vi "Config.vi"(8 "error in (no error)":errorcluster, 10 "Setting":variant, 11 "NI-Sync in":refnum<class "NI-Sync.lvclass">) -> (0 "error out":errorcluster, 3 "NI-Sync out":refnum<class "NI-Sync.lvclass">)   [LabVIEW 2025, in "Synchronization.lvlib" / "NI-Sync.lvclass"]
uses:
  NI-Sync.lvclass
  C:/Users/Public/Documents/Sandia National Labs/TSS Plugin/CEF.lvlibp/Node/CEF_Node.lvclass
  C:/Working copy/tss/Plugin/Engines/Synchronization/Synchronization Instrument/Synchronization Instrument.lvclass
  Synchronization configuration/Synchronization configuration.lvclass
  Synchronization configuration/Synchronization configuration.lvclass/Synchronization configuration.ctl
  NI-Sync.lvclass/NI-Sync.ctl
  Synchronization Channel/Synchronization Channel.lvclass
  Synchronization Channel configuration/Synchronization Channel configuration.lvclass
  C:/Users/Public/Documents/Sandia National Labs/TSS Plugin/Abstract Engine.lvlibp/Plugin/Abstract/Channel configuration/Channel configuration.lvclass
  Synchronization Channel configuration/Synchronization Channel configuration.lvclass/Synchronization Channel configuration.ctl
  Synchronization Channel configuration/Read Sync Channel Setting.vi
  Synchronization configuration/Read Sync Instrument Setting.vi
  Users/Public/Documents/Sandia National Labs/TSS Plugin/CEF.lvlibp/Node/ReadChildren.vi
  Users/Public/Documents/Sandia National Labs/TSS Plugin/Abstract Engine.lvlibp/Plugin/Abstract/Channel configuration/Read Channel Setting.vi
  Users/Public/Documents/Sandia National Labs/TSS Plugin/CEF.lvlibp/Node/CEF_Node.lvclass
  Users/Public/Documents/Sandia National Labs/TSS Plugin/CEF.lvlibp/serializable configuration/CEF_serializable configuration.lvclass
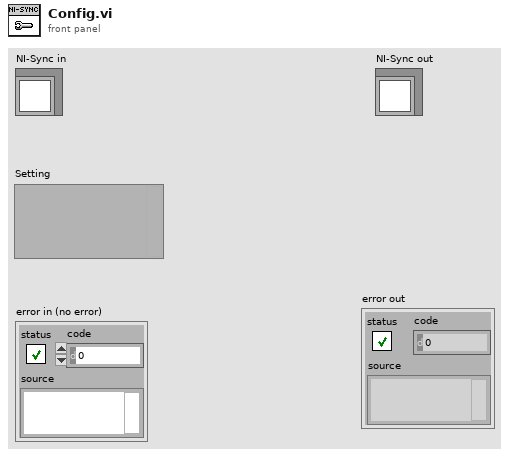
[diagram p1: front panel]
types:
  T1 = typedef "Synchronization.lvlib/Synchronization configuration.lvclass/Sync Instrument Setting.ctl" = cluster{"Synchronization Clock":string, "DDS Clock":dbl, "SyncDivide1":string, "SyncDivide2":string}
  T2 = typedef "Synchronization.lvlib/Synchronization Channel configuration.lvclass/Sync Channel Setting.ctl" = cluster{"Inverter":bool, "Update Edge":string, "Source":string, "Type":string, "Synchronization Clock":string, "Destination":string}
  T3 = typedef "Abstract Engine.lvlibp/Channel configuration.lvclass/Default Channel.ctl" = cluster{"Address":string, "SW Alias":string, "Enabled":bool, "Type":string, "Description":string}
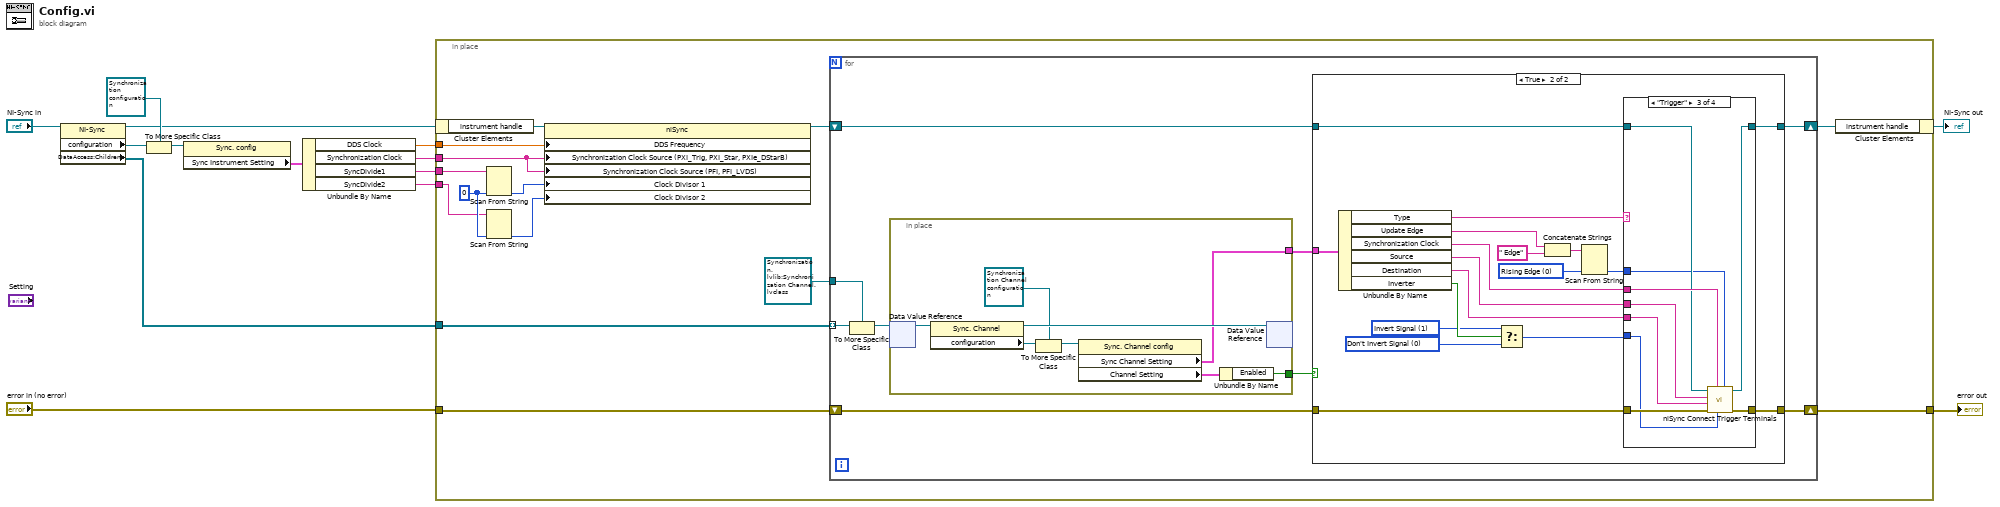
[diagram p0: block diagram]
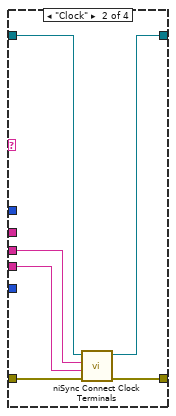
[diagram p4: hidden frame]
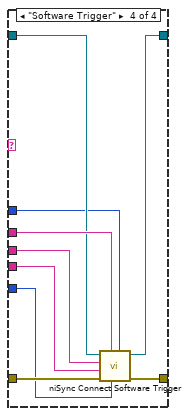
[diagram p5: hidden frame]
diagram:
  n1 = property class="NI-Sync"(reference="NI-Sync in") -> (reference out=w11:refnum<class "NI-Sync.lvclass">, "configuration"=w4:refnum<class "CEF_serializable configuration.lvclass">, "DataAccess:Children"=w2:refnum<data-value>[])  [unwired: 1 in, 1 out]
  n2 = To More Specific Class(target class=refnum<class "Synchronization configuration.lvclass"> refnum ("DMM.lvlib:DMM configuration.lvclass"), reference=w4) -> (specific class reference=w14:refnum<class "Synchronization configuration.lvclass">)  [unwired: 1 in, 1 out]
  n3 = property class="Sync. config"(reference=w14) -> ("Sync Instrument Setting"=w3:T1)  [unwired: 1 in, 2 out]
  n4 = Unbundle By Name(w3) -> ("DDS Clock"=w9:dbl, "Synchronization Clock"=w8:string, "SyncDivide1"=w7:string, "SyncDivide2"=w6:string)
  n5 = in-place {
    in-place-border: w9 -> [w28]
    in-place-border: w8 -> [w27]
    in-place-border: w7 -> [w26]
    in-place-border: w6 -> [w23]
    in-place-border: w2 -> [w17]
    in-place-border: [w19] -> w5
    in-place-border: "error in (no error)" -> [w15]
    w24 = 0 ("Synchronization Clock Properties:Clock Divisor 1")
    n6 = in-place-cluster #1(w11) -> ("instrument handle"=w16:refnum<k15>)
    n7 = Scan From String(input string=w26, default 1=w24) -> (output 1=w25:i32)  [unwired: 3 in, 3 out]
    n8 = Scan From String(input string=w23, default 1=w24) -> (output 1=w22:i32)  [unwired: 3 in, 3 out]
    n9 = property class="niSync"(reference=w16, "DDS Frequency"=w28, "Synchronization Clock Source (PXI_Trig, PXI_Star, PXIe_DStarB)"=w27, "Synchronization Clock Source (PFI, PFI_LVDS)"=w27, "Clock Divisor 1"=w25, "Clock Divisor 2"=w22) -> (reference out=w21:refnum<k15>)  [unwired: 1 in, 1 out]
    n10 = for {
      shift-right: [w35] -> w19
      shift-left: w15 -> [w36]
      shift-right: [w34] -> w20
      shift-left: w21 -> [w37]
      tunnel: refnum<data-value> refnum ("data value reference") -> [w33]
      tunnel: w17 -> [w32] mode=indexing
      n11 = To More Specific Class(target class=w33, reference=w32) -> (specific class reference=w31:refnum<data-value>)  [unwired: 1 in, 1 out]
      n12 = in-place {
        in-place-border: [w40] -> w30
        in-place-border: [w38] -> w29
        # "Initialize the front panel controls when loaded"
        n13 = in-place-dvr #2(w31) -> (w45:refnum<class "Synchronization Channel.lvclass">)  [unwired: 1 out]
        n14 = property class="Sync. Channel"(reference=w45) -> (reference out=w44:refnum<class "Synchronization Channel.lvclass">, "configuration"=w43:refnum<class "CEF_serializable configuration.lvclass">)  [unwired: 1 in, 1 out]
        n15 = To More Specific Class(target class=refnum<class "Synchronization Channel configuration.lvclass"> refnum ("Synchronization.lvlib:Synchronization Channel configuration.lvclass"), reference=w43) -> (specific class reference=w41:refnum<class "Synchronization Channel configuration.lvclass">)  [unwired: 1 in, 1 out]
        n16 = property class="Sync. Channel config"(reference=w41) -> ("Sync Channel Setting"=w38:T2, "Channel Setting"=w39:T3)  [unwired: 1 in, 2 out]
        n17 = Unbundle By Name(w39) -> ("Enabled"=w40:bool)
        n18 = in-place-dvr #2(w44) -> ()  [unwired: 2 out]
      }
      n19 = case shown="True" w30 {
        tunnel: w37 -> [w46 w64]
        tunnel: w36 -> [w47 w59]
        tunnel: [w47 w58] -> w35
        tunnel: [w46 w54] -> w34
        tunnel: w29 -> [_ w53]
        frame False {
        }
        frame True {
          w49 = 0 items=["Rising Edge", "Falling Edge"] ("update edge (Rising Edge)")
          w56 = 1 items=["Don't Invert Signal", "Invert Signal"] ("invert (Don't Invert Signal)")
          w57 = 0 items=["Don't Invert Signal", "Invert Signal"] ("invert (Don't Invert Signal)")
          n20 = Unbundle By Name(w53) -> ("Type"=w65:string, "Update Edge"=w52:string, "Synchronization Clock"=w63:string, "Source"=w62:string, "Destination"=w61:string, "Inverter"=w60:bool)
          n21 = Select(t=w56, s=w60, f=w57) -> (s? t:f=w55:i32)
          n22 = Concatenate Strings(w52, " Edge" ("string")) -> (w50:string)
          n23 = Scan From String(input string=w50, default 1=w49) -> (output 1=w48:i32)  [unwired: 3 in, 3 out]
          n24 = case shown="\"Trigger\"" w65 {
            tunnel: w64 -> [w66 w73 w76 w85]
            tunnel: w63 -> [_ _ w79 w89]
            tunnel: w62 -> [_ w72 w78 w88]
            tunnel: w61 -> [_ w71 w77 w87]
            tunnel: w59 -> [w67 w70 w82 w91]
            tunnel: [w67 w69 w81 w90] -> w58
            tunnel: w55 -> [_ _ w80 w86]
            tunnel: [w66 w68 w75 w84] -> w54
            tunnel: w48 -> [_ _ w74 w83]
            frame "None", Default {
            }
            frame "Clock" {
              n25 = call <instrlib>:"niSync Connect Clock Terminals.vi"("error in (no error)"=w70, "destination terminal"=w71, "source terminal"=w72, "instrument handle"=w73) -> ("error out"=w69:errorcluster, "instrument handle out"=w68:refnum<k15>)  [unwired: 6 in]
            }
            frame "Trigger" {
              n26 = call <instrlib>:"niSync Connect Trigger Terminals.vi"("update edge (Rising Edge)"=w74, "invert (Don't Invert Signal)"=w80, "synchronization clock"=w79, "error in (no error)"=w82, "destination terminal"=w77, "source terminal"=w78, "instrument handle"=w76) -> ("error out"=w81:errorcluster, "instrument handle out"=w75:refnum<k15>)  [unwired: 3 in]
            }
            frame "Software Trigger" {
              n27 = call <instrlib>:"niSync Connect Software Trigger.vi"("update edge (Rising Edge)"=w83, "invert (Don't Invert Signal)"=w86, "synchronization clock"=w89, "error in (no error)"=w91, "destination terminal"=w87, "source terminal"=w88, "instrument handle"=w85) -> ("error out"=w90:errorcluster, "instrument handle out"=w84:refnum<k15>)  [unwired: 3 in]
            }
          }
        }
      }
    }
    n28 = in-place-cluster #1("instrument handle"=w20) -> (→"NI-Sync out":refnum<class "NI-Sync.lvclass">)
  }
  "error out" <- w5
